vi "acquisition test fixed exposure.vi"() -> ()   [LabVIEW 2023]
uses:
  <vilib>/vision/driver/IMAQdx.llb/IMAQdx Attribute Type.ctl
  <vilib>/userDefined/High Color/IMAQdx.ctl
  <vilib>/vision/driver/IMAQdx.llb/IMAQdx Buffer Number Mode.ctl
  <vilib>/DAQmx/write.llb/DAQmx Write (Digital Wfm 1Chan NSamp).vi
  <vilib>/DAQmx/read.llb/DAQmx Read (Analog Wfm 1Chan NSamp).vi
  <extravilib>/ChannelInstances/Tag-bool/Write With Abort.vi
  <extravilib>/ChannelInstances/Tag-bool/Read With Abort.vi
  <vilib>/DAQmx/create/channels.llb/DAQmx Create Channel (AI-Voltage-Basic).vi
  <vilib>/DAQmx/configure/timing.llb/DAQmx Timing (Sample Clock).vi
  <vilib>/DAQmx/create/channels.llb/DAQmx Create Channel (DO-Digital Output).vi
  <vilib>/Waveform/DWDTOps.llb/DWDT Boolean Array to Digital.vi
  <vilib>/DAQmx/create/channels.llb/DAQmx Create Channel (CO-Pulse Generation-Frequency).vi
  <vilib>/DAQmx/configure/timing.llb/DAQmx Timing (Implicit).vi
  <vilib>/Waveform/DWDTOps.llb/DWDT Uncompress Digital.vi
  <vilib>/DAQmx/miscellaneous.llb/DAQmx Fill In Error Info.vi
  <extravilib>/ChannelInstances/Tag-bool/Instantiate.vi
  <extravilib>/ChannelInstances/Tag-bool/EndpointRead.vi
  <extravilib>/ChannelInstances/Tag-bool/Endpoint.vi
  <extravilib>/ChannelInstances/Tag-bool.lvlib
  <vilib>/vision/driver/NI_Vision_Acquisition_Software.lvlib
  <resource>/objmgr/imaqdx.rc
panel:
  out "digital waveform":digitalwaveform(waveform)={"t0"=timestamp(0 s since 1904-01-01), "dt"=1.0, "Y"={"transitions"=[], "data"=[]}}
  out "Attribute Information":T2
  out "error out":errorcluster
  out "ValueDBL":dbl
  out "Attribute Information Array 2":T3(array[cluster])
  out "Images Missed":u32
  out "Images Behind":i32
  out "Processed Frames per Second":dbl
  out "Acquired Frames per Second":dbl
  out "Image":T4(plugin-control)
  out "Waveform Chart":waveform(dbl)(graph)
  in  "stop":bool
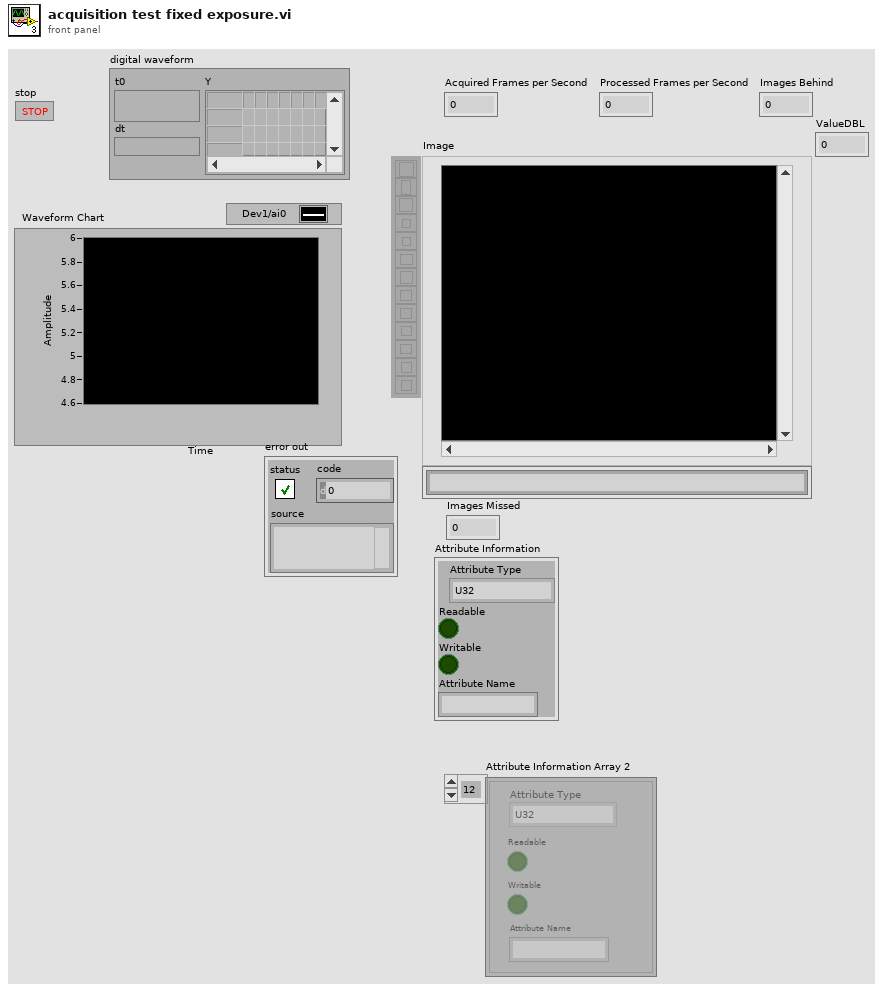
[diagram p1: front panel]
types:
  T1 = typedef "NI_Vision_Acquisition_Software.lvlib/IMAQdx Attribute Type.ctl" = enum32{"U32", "I64", "DBL", "String", "Enum", "Bool", "Command"}
  T2 = cluster{"Attribute Type":T1, "Readable":bool, "Writable":bool, "Attribute Name":string}
  T3 = cluster{"Attribute Type":T1, "Readable":bool, "Writable":bool, "Attribute Name":string}[]
  T4 = typedef "IMAQ Image.ctl" = refnum<image>
  T5 = typedef "IMAQdx.ctl" = refnum<k21>
  T6 = typedef "Tag-bool.lvlib/))Channel.ctl" = refnum<queue>
  T7 = typedef "NI_Vision_Acquisition_Software.lvlib/IMAQdx Buffer Number Mode.ctl" = enum32{"Next", "Last", "Buffer Number", "Every", "Last New"}
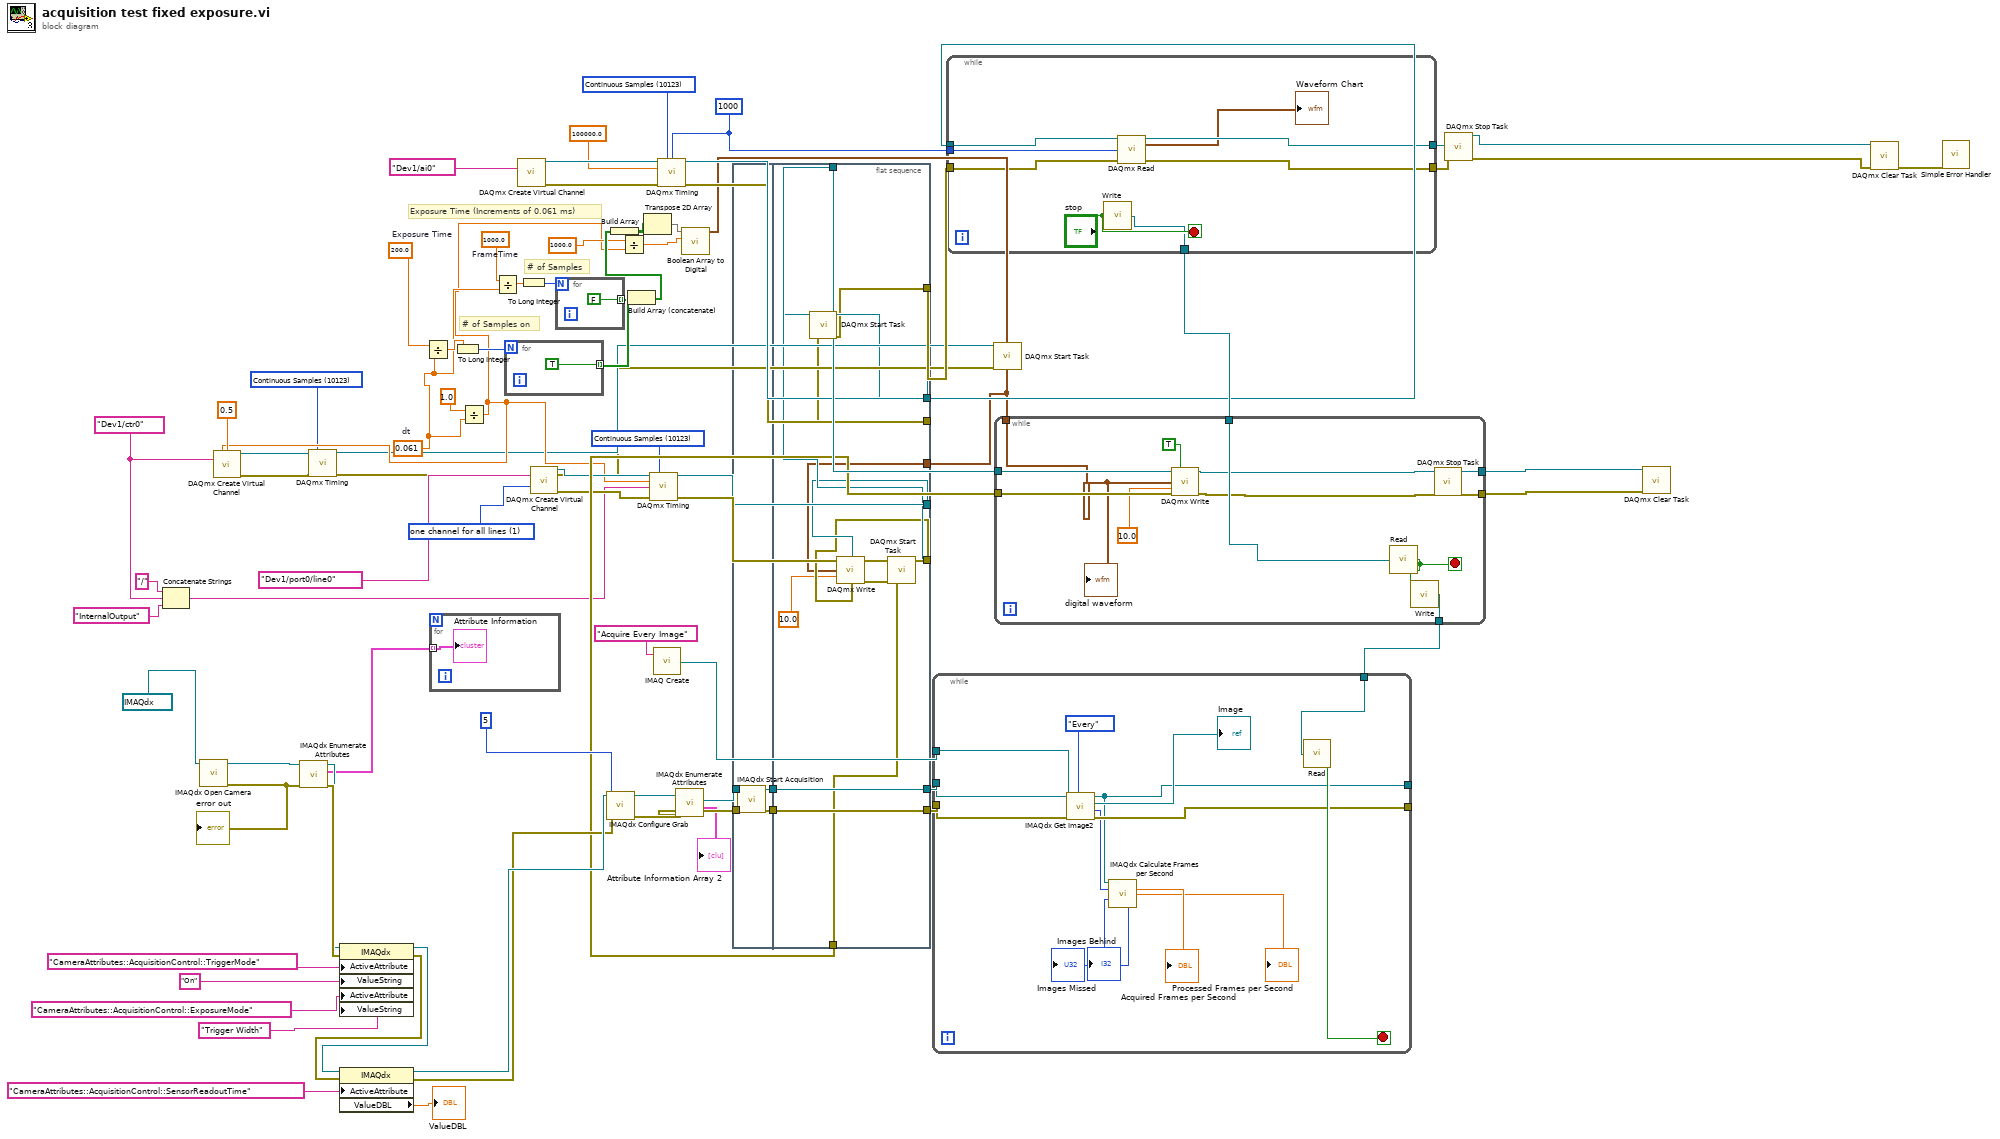
[diagram p0: block diagram]
diagram:
  w8 = 10123 items=["Finite Samples"=10178, "Continuous Samples"=10123, "Hardware Timed Single Point"=12522] ("sample mode")
  w13 = 10123 items=["Finite Samples"=10178, "Continuous Samples"=10123, "Hardware Timed Single Point"=12522] ("sample mode")
  w22 = 1 items=["one channel for each line", "one channel for all lines"] ("line grouping")
  w32 = 1000.0  # FrameTime
  w23 = 0.061  # dt
  w41 = 200.0  # Exposure Time
  w78 = 10123 items=["Finite Samples"=10178, "Continuous Samples"=10123, "Hardware Timed Single Point"=12522] ("sample mode")
  w79 = 1000 ("number of samples per channel")
  w5 = tag "Dev1/ctr0" ("counter")
  # "# of Samples on"
  # "# of Samples"
  # "Exposure Time (Increments of 0.061 ms)"
  n1 = Concatenate Strings("/", w5, "InternalOutput" ("string")) -> (w4:string)
  n2 = call <vilib>:"IMAQdx Open Camera.vi"("Session In"=T5 "cam0") -> ("error out"=w55:errorcluster, "Session Out"=w67:T5)  [unwired: 9 in]
  "error out" <- w55
  n3 = call <vilib>:"IMAQdx Enumerate Attributes.vi"("error in"=w55, "Session In"=w67) -> ("error out"=w66:errorcluster, "Attribute Information Array"=w50:T3, "Session Out"=w65:T5)  [unwired: 7 in]
  n4 = property class="IMAQdx"(reference=w65, error in=w66, "ActiveAttribute"="CameraAttributes::AcquisitionControl::TriggerMode", "ValueString"="On", "ActiveAttribute"="CameraAttributes::AcquisitionControl::ExposureMode", "ValueString"="Trigger Width") -> (reference out=w52:T5, error out=w51:errorcluster)
  n5 = property class="IMAQdx"(reference=w52, error in=w51, "ActiveAttribute"="CameraAttributes::AcquisitionControl::SensorReadoutTime") -> (reference out=w59:T5, error out=w58:errorcluster, "ValueDBL"=→"ValueDBL":dbl)
  n6 = Divide(x=w41, y=w23) -> (x/y=w31:dbl)
  n7 = for {
    tunnel: w50 -> [w86] mode=indexing
    "Attribute Information" <- w86
  }
  n8 = To Long Integer(number=w31) -> (32bit integer=w30:i32)
  n9 = Divide(x=1.0, y=w23) -> (x/y=w9:dbl)
  n10 = call-poly <vilib>:"DAQmx Create Virtual Channel.vi"("frequency"=w9, "duty cycle"=0.5, "counter"=w5) -> ("task out"=w12:refnum<k21>, "error out"=w11:errorcluster)  [unwired: 11 in]
  n11 = call-poly <vilib>:"DAQmx Timing.vi"("task/channels in"=w12, "sample mode"=w8, "error in"=w11) -> ("task out"=w3:refnum<k21>, "error out"=w2:errorcluster)  [unwired: 11 in]
  n12 = Divide(x=w32, y=w23) -> (x/y=w29:dbl)
  n13 = for {
    N: w30 -> [_]
    tunnel: [TRUE] -> w27 mode=indexing
  }
  n14 = call-poly <vilib>:"DAQmx Create Virtual Channel.vi"("physical channels"=tag "Dev1/ai0") -> ("task out"=w85:refnum<k21>, "error out"=w84:errorcluster)  [unwired: 13 in]
  n15 = To Long Integer(number=w29) -> (32bit integer=w28:i32)
  n16 = call-poly <vilib>:"DAQmx Create Virtual Channel.vi"("lines"=tag "Dev1/port0/line0", "line grouping"=w22) -> ("task out"=w17:refnum<k21>, "error out"=w16:errorcluster)  [unwired: 12 in]
  n17 = for {
    N: w28 -> [_]
    tunnel: [FALSE] -> w26 mode=indexing
  }
  n18 = call <vilib>:"IMAQdx Configure Grab.vi"("error in"=w58, "Number of Buffers"=u32 5, "Session In"=w59) -> ("error out"=w63:errorcluster, "Session Out"=w64:T5)  [unwired: 7 in]
  n19 = Divide(x=1000.0 ("y"), y=w9) -> (x/y=w19:dbl)
  n20 = Build Array (concatenate)(w27, w26) -> (w25:bool[])
  n21 = Build Array(w25) -> (w21:bool[][])
  n22 = Transpose 2D Array(2D array=w21) -> (transposed array=w20:bool[][])
  n23 = call-poly <vilib>:"DAQmx Timing.vi"("task/channels in"=w17, "sample mode"=w13, "rate"=w9, "source"=w4, "error in"=w16) -> ("task out"=w14:refnum<k21>, "error out"=w15:errorcluster)  [unwired: 9 in]
  n24 = call "IMAQ Create"("Image Name"="Acquire Every Image") -> ("New Image"=w71:T4)  [unwired: 3 in, 2 out]
  n25 = call-poly <vilib>:"DAQmx Timing.vi"("task/channels in"=w85, "sample mode"=w78, "samples per channel"=w79, "rate"=100000.0, "error in"=w84) -> ("task out"=w36:refnum<k21>, "error out"=w35:errorcluster)  [unwired: 9 in]
  n26 = call <vilib>:"IMAQdx Enumerate Attributes.vi"("error in"=w63, "Session In"=w64) -> ("error out"=w61:errorcluster, "Attribute Information Array"=→"Attribute Information Array 2":T3, "Session Out"=w62:T5)  [unwired: 7 in]
  n27 = call-poly <vilib>:"Boolean Array to Digital.vi"("sample rate"=w19, "boolean array"=w20) -> ("digital waveform"=w1:digitalwaveform)  [unwired: 8 in, 1 out]
  n28 = flat-sequence {
    tunnel: w62 -> [w90]
    tunnel: w61 -> [w89]
    tunnel: [w92] -> w40
    tunnel: [w91] -> w39
    tunnel: [w105] -> w73
    tunnel: [w106] -> w74
    tunnel: w40 -> [w106]
    tunnel: w39 -> [w105]
    tunnel: [w104] -> w38
    tunnel: [w103] -> w37
    tunnel: w36 -> [w102]
    tunnel: w35 -> [w101]
    tunnel: [w100] -> w34
    tunnel: [w99] -> w33
    tunnel: w15 -> [w96]
    tunnel: w14 -> [w98]
    tunnel: w1 -> [w94]
    frame #0 {
      n29 = call <vilib>:"IMAQdx Start Acquisition.vi"("error in"=w89, "Session In"=w90) -> ("error out"=w91:errorcluster, "Session Out"=w92:T5)  [unwired: 8 in]
    }
    frame #1 {
      n30 = call <vilib>:"DAQmx Start Task.vi"("task/channels in"=w102, "error in"=w101) -> ("task out"=w100:refnum<k21>, "error out"=w99:errorcluster)  [unwired: 12 in]
      n31 = call-poly <vilib>:"DAQmx Write.vi"("task/channels in"=w98, "data"=w94, "timeout"=10.0, "error in"=w96) -> ("task out"=w97:refnum<k21>, "error out"=w95:errorcluster)  [unwired: 9 in, 1 out]
      n32 = call <vilib>:"DAQmx Start Task.vi"("task/channels in"=w97, "error in"=w95) -> ("task out"=w104:refnum<k21>, "error out"=w103:errorcluster)  [unwired: 12 in]
    }
  }
  n33 = while {
    tunnel: [w114] -> w45
    tunnel: [w113] -> w44
    tunnel: w34 -> [w112]
    tunnel: w33 -> [w111]
    tunnel: w79 -> [w110]
    tunnel: [w107] -> w77
    stop <- "stop" stop-if-true
    n34 = call <extravilib>:"Write.vi"("element"="stop") -> ("channel"=w107:T6)  [unwired: 1 out]
    n35 = call-poly <vilib>:"DAQmx Read.vi"("task/channels in"=w112, "number of samples per channel"=w110, "error in"=w111) -> ("task out"=w114:refnum<k21>, "data"=→"Waveform Chart":waveform(dbl), "error out"=w113:errorcluster)  [unwired: 10 in]
  }
  n36 = call <vilib>:"DAQmx Start Task.vi"("task/channels in"=w3, "error in"=w2) -> ()  [unwired: 12 in, 2 out]
  n37 = while {
    tunnel: [w118] -> w49
    tunnel: [w119] -> w48
    tunnel: w38 -> [w124]
    tunnel: w37 -> [w123]
    tunnel: w77 -> [w122]
    tunnel: [w120] -> w76
    tunnel: w1 -> [w117]
    stop <- w121 stop-if-true
    n38 = call-poly <vilib>:"DAQmx Write.vi"("task/channels in"=w124, "auto start"=TRUE, "data"=w117, "timeout"=10.0, "error in"=w123) -> ("task out"=w118:refnum<k21>, "error out"=w119:errorcluster)  [unwired: 8 in, 1 out]
    n39 = call <extravilib>:"Read.vi"("channel"=w122) -> ("element"=w121:bool)  [unwired: 1 in, 1 out]
    n40 = call <extravilib>:"Write.vi"("element"=w121) -> ("channel"=w120:T6)  [unwired: 1 out]
    "digital waveform" <- w117
  }
  n41 = while {
    tunnel: w76 -> [w138]
    tunnel: w74 -> [w136]
    tunnel: w73 -> [w135]
    tunnel: [w130] -> _
    tunnel: [w134] -> _
    tunnel: w71 -> [w132]
    stop <- w137 stop-if-true
    n42 = call <vilib>:"IMAQdx Get Image2.vi"("Buffer Number Mode (Next)"=IMAQdx_Buffer_Number_Mode."Every", "error in"=w135, "Image In"=w132, "Session In"=w136) -> ("error out"=w134:errorcluster, "Buffer Number Out"=w129:u32, "Image Out"=→"Image":T4, "Session Out"=w130:T5)  [unwired: 4 in]
    n43 = call <vilib>:"IMAQdx Calculate Frames per Second.vi"("Session In"=w130, "Buffer Number"=w129) -> ("Acquired Frames per Second"=→"Acquired Frames per Second":dbl, "Processed Frames per Second"=→"Processed Frames per Second":dbl, "Images Behind"=→"Images Behind":i32, "Images Missed"=→"Images Missed":u32)  [unwired: 7 in, 3 out]
    n44 = call <extravilib>:"Read.vi"("channel"=w138) -> ("element"=w137:bool)  [unwired: 1 in, 1 out]
  }
  n45 = call <vilib>:"DAQmx Stop Task.vi"("task/channels in"=w49, "error in"=w48) -> ("task out"=w47:refnum<k21>, "error out"=w46:errorcluster)  [unwired: 12 in]
  n46 = call <vilib>:"DAQmx Stop Task.vi"("task/channels in"=w45, "error in"=w44) -> ("task out"=w43:refnum<k21>, "error out"=w42:errorcluster)  [unwired: 12 in]
  n47 = call <vilib>:"DAQmx Clear Task.vi"("task in"=w47, "error in"=w46) -> ()  [unwired: 13 in, 1 out]
  n48 = call <vilib>:"DAQmx Clear Task.vi"("task in"=w43, "error in"=w42) -> ("error out"=w80:errorcluster)  [unwired: 13 in]
  n49 = call <vilib>:"Simple Error Handler.vi"("error in (no error)"=w80) -> ()  [unwired: 4 in, 5 out]
